vi "PictureData.vi"(11 "picture":picture) -> (0 "Size":T2, 1 "Origin":T1)   [LabVIEW 2016, in "Dxf.lvlib"]
uses:
  <vilib>/Utility/miscctls.llb/LVBoundsTypeDef.ctl
  <vilib>/Utility/miscctls.llb/LVPointTypeDef.ctl
  Dxf.lvlib
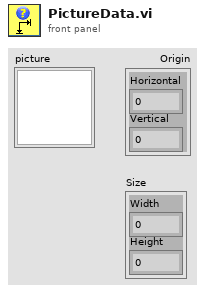
[diagram p1: front panel]
types:
  T1 = typedef "LVPointTypeDef.ctl" = cluster{"Horizontal":i16, "Vertical":i16}
  T2 = typedef "LVBoundsTypeDef.ctl" = cluster{"Width":u32, "Height":u32}
  T3 = typedef "imagedata.ctl" = cluster{"image type":i32, "image depth":i32, "image":u8[], "mask":u8[], "colors":u32[], "Rectangle":cluster{"left":i16, "top":i16, "right":i16, "bottom":i16}}
  T4 = cluster{"left":i16, "top":i16, "right":i16, "bottom":i16}
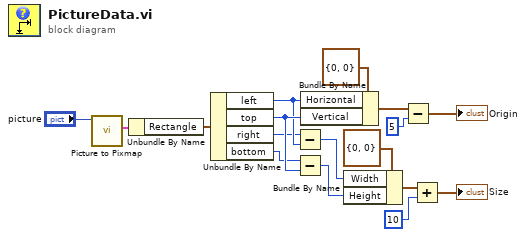
[diagram p0: block diagram]
diagram:
  n1 = call <vilib>:"Picture to Pixmap.vi"("picture"="picture") -> ("image data"=w2:T3)  [unwired: 9 in, 1 out]
  n2 = Unbundle By Name(w2) -> ("Rectangle"=w4:T4)
  n3 = Unbundle By Name(w4) -> ("left"=w7:i16, "top"=w9:i16, "right"=w6:i16, "bottom"=w8:i16)
  n4 = Subtract(x=w6, y=w7) -> (x-y=w10:i16)
  n5 = Subtract(x=w8, y=w9) -> (x-y=w11:i16)
  n6 = Bundle By Name(cluster=T1 {"Horizontal"=0, "Vertical"=0} ("Origin"), "Horizontal"=w7, "Vertical"=w9) -> (w12:T1)
  n7 = Bundle By Name(cluster=T2 {"Width"=0, "Height"=0} ("XControl:Container Bounds"), "Width"=w10, "Height"=w11) -> (w14:T2)
  n8 = Subtract(x=w12, y=i16 5) -> (x-y=→"Origin":T1)
  n9 = Add(x=w14, y=u32 10) -> (x+y=→"Size":T2)
